vi "hash.vi"(11 "input":i64) -> (3 "output":i64)   [LabVIEW 2015]
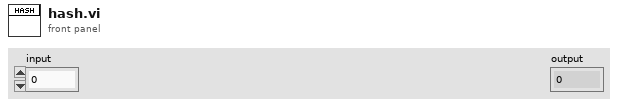
[diagram p1: front panel]
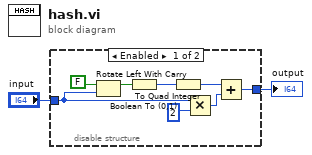
[diagram p0: block diagram]
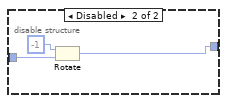
[diagram p2: hidden frame]
diagram:
  n1 = disable-structure shown="Enabled" {
    disable-tunnel: "input" -> [w4 w13]
    disable-tunnel: [w3 w11] -> w1
    frame Enabled {
      n2 = Rotate Left With Carry(2:w4, 3:FALSE ("carry")) -> (1:w8:bool)  [unwired: 1 out]
      n3 = Boolean To (0,1)(Boolean=w8) -> (0, 1=w7:i16)
      n4 = To Quad Integer(1:w7) -> (0:w5:i64)
      n5 = Multiply(x=w4, y=i64 2) -> (x*y=w6:i64)
      n6 = Add(x=w5, y=w6) -> (x+y=w3:i64)
    }
    frame Disabled {
      n7 = Rotate(1:w13, 2:i16 -1 ("y")) -> (0:w11:i64)
    }
  }
  "output" <- w1
